vi "Tektronix TDS 200 1000 2000 Series Acquire FFT Waveform.vi"() -> ()   [LabVIEW 2012]
doc: "This example shows how to use autosetup and acquire a waveform on a FFT channel."
uses:
  <instrlib>/Tektronix TDS 200 1000 2000 Series/Public/Data/Read (Single Waveform).vi
  <instrlib>/Tektronix TDS 200 1000 2000 Series/Tektronix TDS 200 1000 2000 Series.lvlib
panel:
  in  "Enable Display (T: Enable)":bool=TRUE
  in  "FFT Window (0: Hanning)":i32(ring) items=["Hanning", "Flattop", "Rectangular"]
  in  "FFT Channel (0: Channel 1)":i32(ring) items=["Channel 1", "Channel 2"]
  in  "Serial Configuration":T1={"Baud Rate"=9600, "Parity"=0, "Stop Bits"=10, "Flow Control"=0} {"Flow Control" items=["None", "XON/XOFF", "RTS/CTS", "XON/XOFF & RTS/CTS", "DTR/DSR", "XON/XOFF & DTR/DSR"]; "Stop Bits" items=["1.0"=10, "1.5"=15, "2.0"=20]; "Parity" items=["None", "Odd", "Even", "Mark", "Space"]; "Baud Rate" items=["300"=300, "600"=600, "1200"=1200, "2400"=2400, "4800"=4800, "9600"=9600, "19200"=19200]}
  in  "Probe Attenuation (10.0)":dbl=10.0
  in  "Timeout (10000 ms)":u32=10000
  out "Waveform Data":waveform(dbl)(graph)
  in  "VISA resource name":refnum<visa-resource-name>
  # "(C) 2014 National Instruments.  ALL RIGHTS RESERVED."
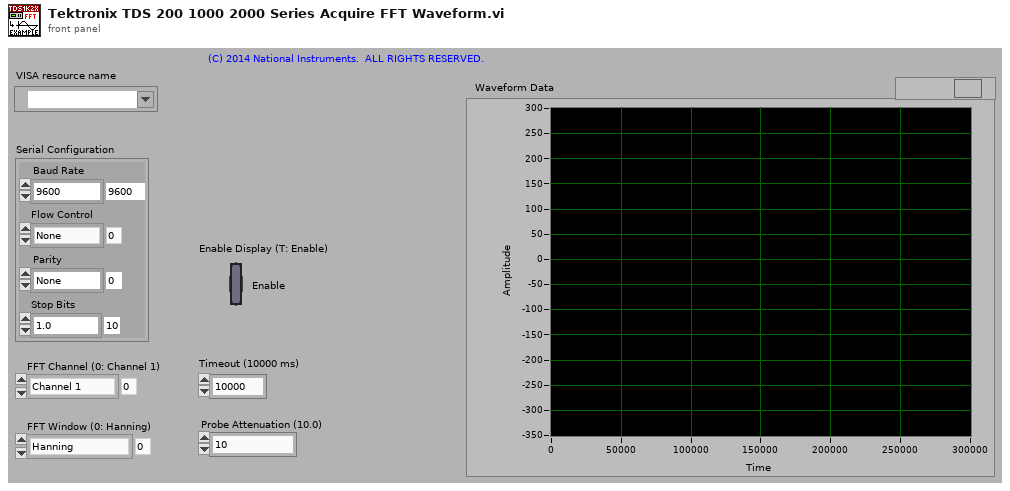
[diagram p1: front panel]
types:
  T1 = cluster{"Baud Rate":u32, "Parity":u16, "Stop Bits":u16, "Flow Control":u16}
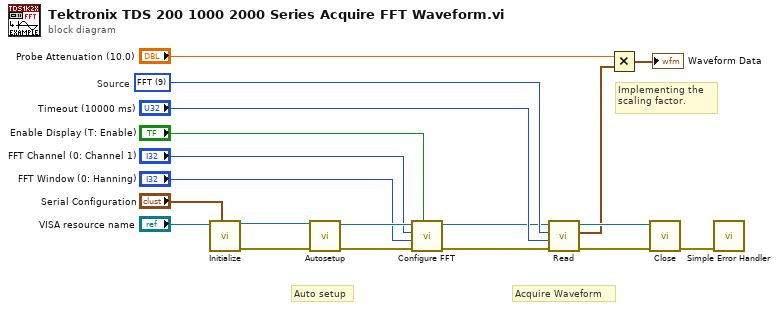
[diagram p0: block diagram]
diagram:
  w8 = u16 9 items=["Channel 1", "Channel 2", "Channel 3", "Channel 4", "Math", "Reference A", "Reference B", "Reference C", "Reference D", "FFT"]  # Source
  # "Implementing the \nscaling factor."
  # "Acquire Waveform"
  # "Auto setup"
  n1 = call <instrlib>:"Initialize.vi"("Serial Configuration"="Serial Configuration", "VISA resource name"="VISA resource name") -> ("error out"=w15:errorcluster, "VISA resource name out"=w14:refnum<visa-resource-name>)  [unwired: 3 in, 5 out]
  n2 = call <instrlib>:"Autosetup.vi"("error in (no error)"=w15, "VISA resource name"=w14) -> ("error out"=w7:errorcluster, "VISA resource name out"=w6:refnum<visa-resource-name>)  [unwired: 8 out]
  n3 = call <instrlib>:"Configure FFT.vi"("Enable FFT Display (T: Enable)"="Enable Display (T: Enable)", "error in (no error)"=w7, "FFT Window (0: Hanning)"="FFT Window (0: Hanning)", "FFT Channel (0: Channel 1)"="FFT Channel (0: Channel 1)", "VISA resource name"=w6) -> ("error out"=w4:errorcluster, "VISA resource name out"=w5:refnum<visa-resource-name>)  [unwired: 1 in, 4 out]
  n4 = call-poly <instrlib>:"Read.vi"("error in (no error)"=w4, "Timeout (10000 ms)"="Timeout (10000 ms)", "Source (0: Channel 1)"=w8, "VISA resource name"=w5) -> ("error out"=w17:errorcluster, "Waveform Data"=w12:waveform(dbl), "VISA resource name out"=w18:refnum<visa-resource-name>)  [unwired: 5 out]
  n5 = Multiply(x="Probe Attenuation (10.0)", y=w12) -> (x*y=→"Waveform Data":waveform(dbl))
  n6 = call <instrlib>:"Close.vi"("error in (no error)"=w17, "VISA resource name"=w18) -> ("error out"=w19:errorcluster)  [unwired: 9 out]
  n7 = call <vilib>:"Simple Error Handler.vi"("error in (no error)"=w19) -> ()  [unwired: 1 in, 8 out]
